vi "Configure.vi"(8 "error in (no error)":errorcluster, 10 "Parameters":variant, 11 "Output Process in":refnum<class "Random Process.lvclass">) -> (0 "error out":errorcluster, 3 "Output Process out":refnum<class "Random Process.lvclass">)   [LabVIEW 2019, in "TelemetryAsync Engine.lvlib" / "Random Process.lvclass"]
uses:
  Random Process.lvclass
  Parent Classes/Process/Process.lvclass
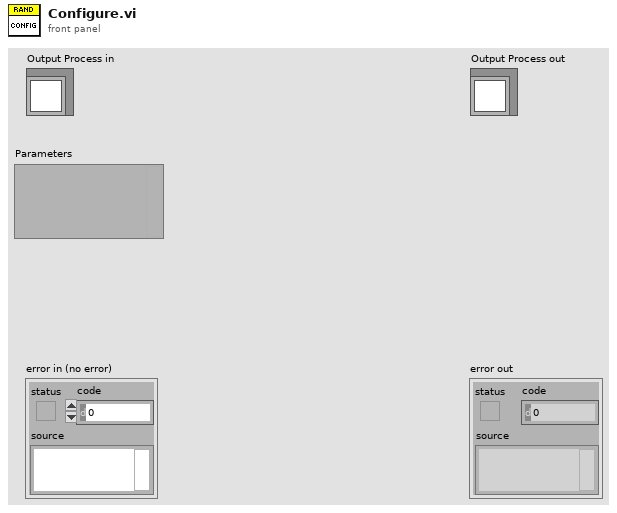
[diagram p1: front panel]
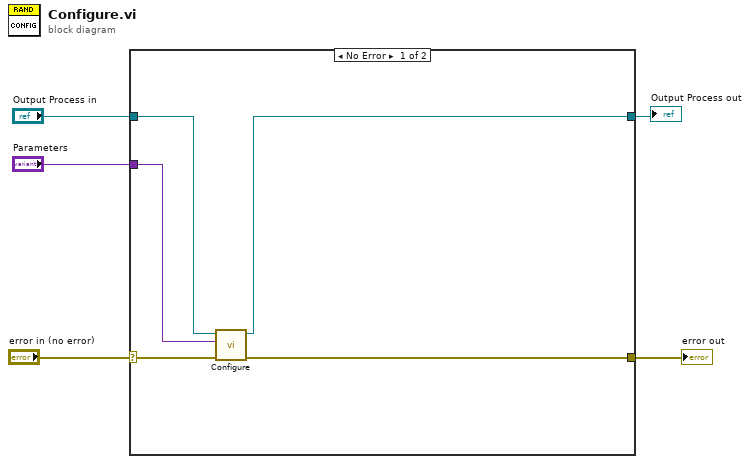
[diagram p0: block diagram]
diagram:
  n1 = case shown="No Error" "error in (no error)" {
    selector: "error in (no error)" -> [w8 w12]
    tunnel: "Parameters" -> [w10 _]
    tunnel: "Output Process in" -> [w9 w11]
    tunnel: [w7 w11] -> w3
    tunnel: [w6 w12] -> w2
    frame No Error {
      n2 = call-parent "Configure.vi"("error in (no error)"=w8, "Parameters"=w10, "Process in"=w9) -> ("error out"=w6:errorcluster, "Process out"=w7:refnum<class "Random Process.lvclass">)  [unwired: 7 in]
    }
    frame Error {
    }
  }
  "error out" <- w2
  "Output Process out" <- w3
